vi "Create.vi"(4 "Log Map in":refnum<class "LogMap.lvclass">, 6 "commandTimeout":i32=-1, 8 "error in (no error)":errorcluster, 10 "object in":refnum<class>, 11 "SqlMapper in":refnum<class "SqlMapper.lvclass">) -> (0 "error out":errorcluster, 1 "id":i32, 2 "object out":refnum<class>, 3 "SqlMapper out":refnum<class "SqlMapper.lvclass">)   [LabVIEW 2020, in "ORM.lvlib" / "LogMap.lvclass"]
uses:
  LogMap.lvclass
  SqlMapper/SqlMapper.lvclass
  TypeMap/TypeMap.lvclass
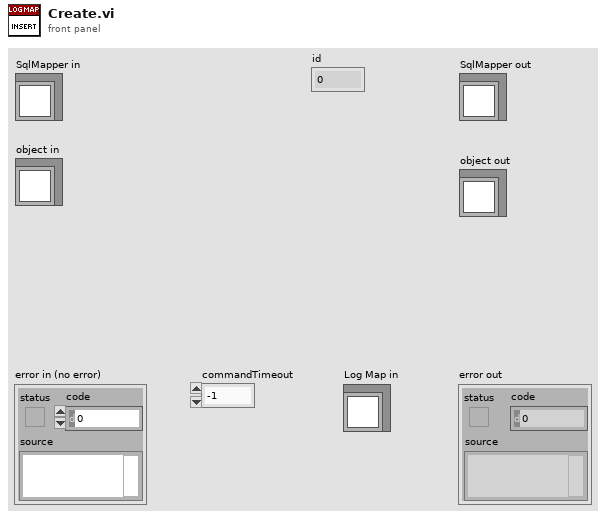
[diagram p1: front panel]
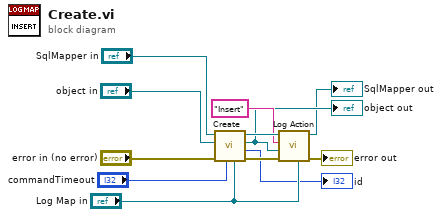
[diagram p0: block diagram]
diagram:
  n1 = call-parent "Create.vi"("TypeMap in"="Log Map in", "commandTimeout"="commandTimeout", "error in (no error)"="error in (no error)", "object in"="object in", "SqlMapper in"="SqlMapper in") -> ("error out"=w5:errorcluster, "id"=→"id":i32, "object out"=w4:refnum<class>, "SqlMapper out"=w8:refnum<class "SqlMapper.lvclass">)  [unwired: 3 in]
  "object out" <- w4
  n2 = call "Log Action.vi"("Log Map in"="Log Map in", "error in (no error)"=w5, "object in"=w4, "ActionType"="Insert", "SqlMapper in"=w8) -> ("error out"=→"error out":errorcluster, "SqlMapper out"=→"SqlMapper out":refnum<class "SqlMapper.lvclass">)  [unwired: 5 in]
